vi "Done.vi"(8 "error in (no error)":errorcluster, 11 "Assembler in":refnum<class "Assembler.lvclass">) -> (0 "error out":errorcluster)   [LabVIEW 2016, in "CLD Exam - ATM.lvlib" / "Assembler.lvclass"]
uses:
  Assembler.lvclass
  Assembler.lvclass/Assembler.ctl
  Log/Text File Sink/Text File Sink.lvclass
  Mediator/Classes/Message Broker Interface Ref/Message Broker Interface Ref.lvclass
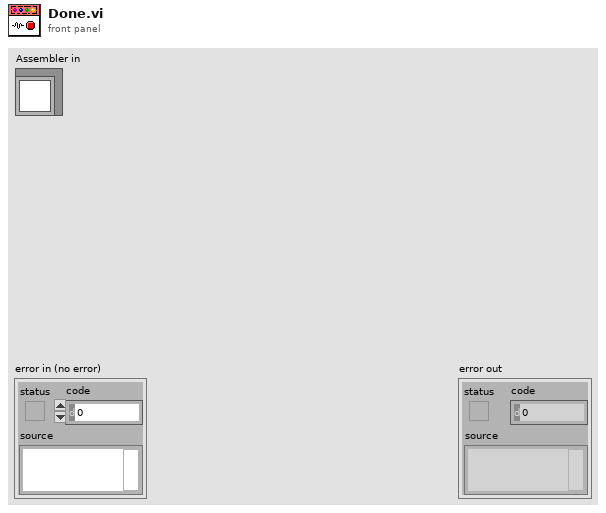
[diagram p1: front panel]
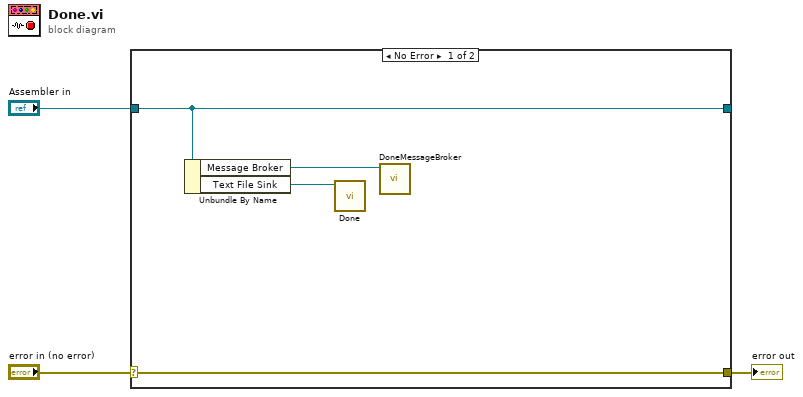
[diagram p0: block diagram]
diagram:
  n1 = case shown="No Error" "error in (no error)" {
    selector: "error in (no error)" -> [w7 w9]
    tunnel: [w7 w9] -> w2
    tunnel: [w6 w8] -> _
    tunnel: "Assembler in" -> [w6 w8]
    frame No Error {
      n2 = Unbundle By Name(w6) -> ("Message Broker"=w5:refnum<class "Message Broker Interface Ref.lvclass">, "Text File Sink"=w4:refnum<class "Text File Sink.lvclass">)
      n3 = call-dynamic "Done.vi"("Text File Sink in"=w4) -> ()  [unwired: 9 in, 2 out]
      n4 = call "DoneMessageBroker.vi"("Message Broker Interface Ref in"=w5) -> ()  [unwired: 9 in, 2 out]
    }
    frame Error {
    }
  }
  "error out" <- w2
